vi "arrays.vi"() -> ()   [LabVIEW 2011]
panel:
  in  "index 1d":dbl
  in  "String":string
  out "String Array":string[](array[string])
  out "element":dbl
  in  "index column controller":dbl
  in  "index row controller":dbl
  in  "Array":dbl[][](array[numeric])
  # "this is a 2d integer array"
  # "index row"
  # "index column"
  # "this is the indicator"
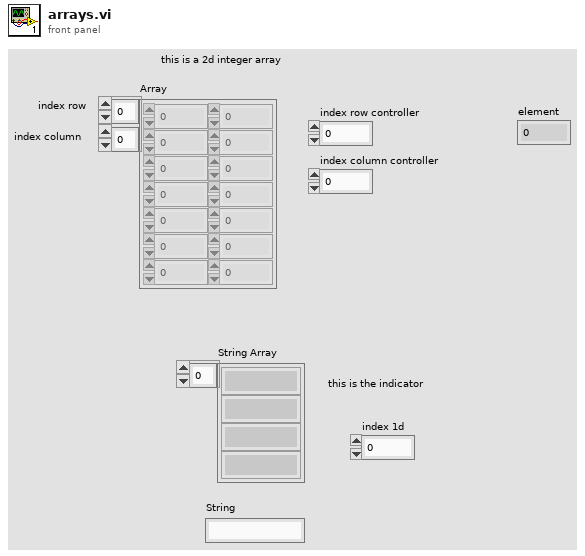
[diagram p1: front panel]
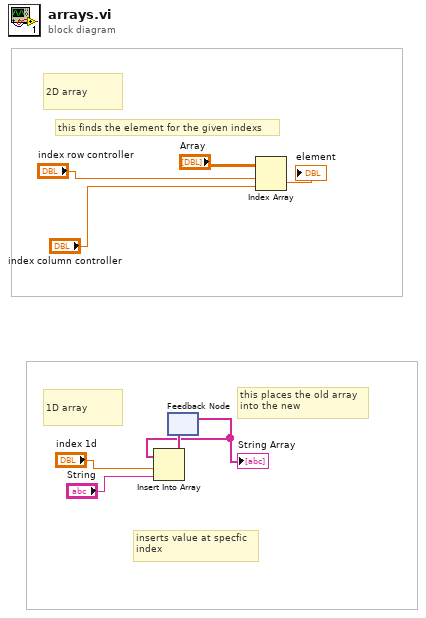
[diagram p0: block diagram]
diagram:
  # "inserts value at specfic \nindex"
  # "this places the old array \ninto the new"
  # "1D array"
  # "2D array"
  # "this finds the element for the given indexs"
  n1 = feedback #1() -> (w3:string[])  [unwired: 1 in]
  "String Array" <- w3
  n2 = Insert Into Array(array=w3, index="index 1d", new element="String") -> (w4:string[])
  n3 = feedback-in #1(w4) -> ()
  n4 = Index Array(array="Array", index (row)="index row controller", index (col)="index column controller") -> (element=→"element":dbl)
